vi "parseCommand.vi"(8 "error in (no error)":errorcluster, 10 "CMDString":string, 11 "CommandParser in":refnum<class "CommandParser.lvclass">) -> (0 "error out":errorcluster, 1 "parameter":variant, 2 "MonoCommand":T1, 3 "CommandParser out":refnum<class "CommandParser.lvclass">)   [LabVIEW 2020, in "CommandParser.lvclass"]
uses:
  CommandParser.lvclass
  Typedefs/MonoCommand.ctl
  Typedefs/wavelength.ctl
  Typedefs/slitWidth.ctl
  Typedefs/GratingType.ctl
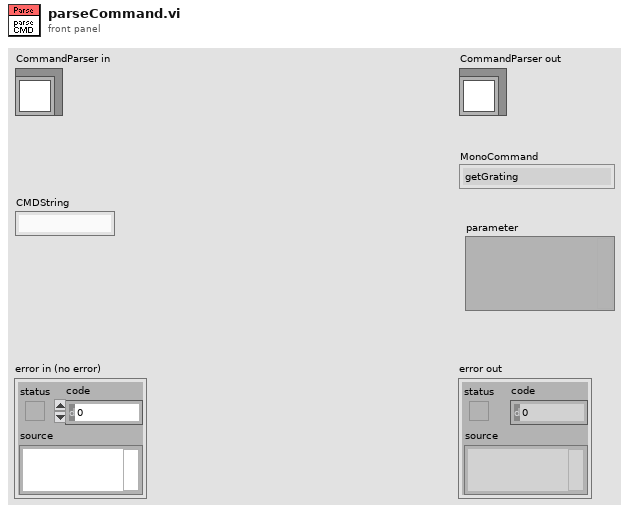
[diagram p1: front panel]
types:
  T1 = typedef "MonoCommand.ctl" = enum16{"getGrating", "getFrontEntranceSlitPosition", "getFrontExitSlitPosition", "getWavelength", "setWavelength", "setGrating", "setFrontEntranceSlitPosition", "setFrontExitSlitPosition", "calibrateWavelength", "getStatus", "Unknown", "reset", "setAll"}
  T2 = typedef "wavelength.ctl" = dbl
  T3 = typedef "slitWidth.ctl" = dbl
  T4 = typedef "GratingType.ctl" = enum16{"Blue", "Red", "Mirror"}
  T5 = cluster{"wavelength":T2, "frontExitSlitWidth":T3, "fronEntranceSlitWidth":T3, "GratingType":T4}
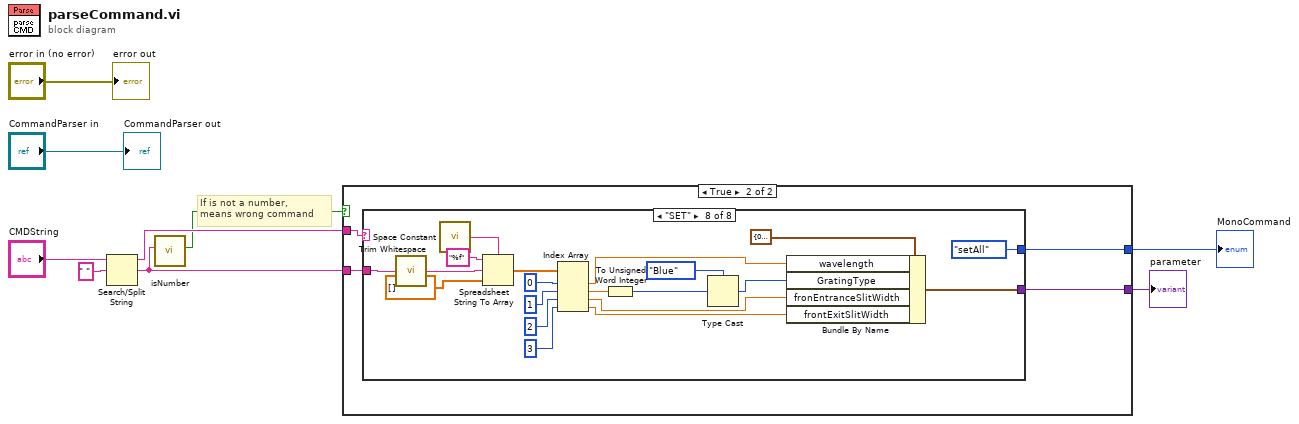
[diagram p0: block diagram]
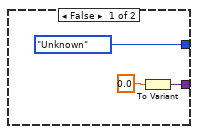
[diagram p2: hidden frame]
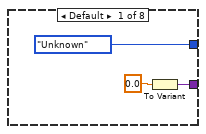
[diagram p3: hidden frame]
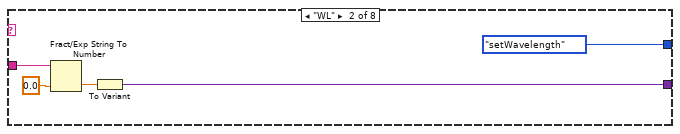
[diagram p4: hidden frame]
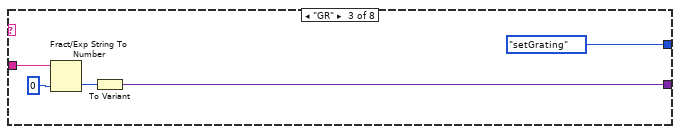
[diagram p5: hidden frame]
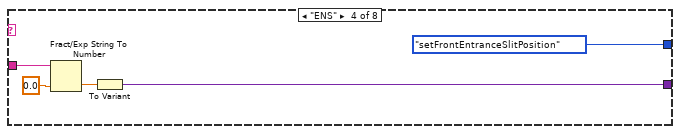
[diagram p6: hidden frame]
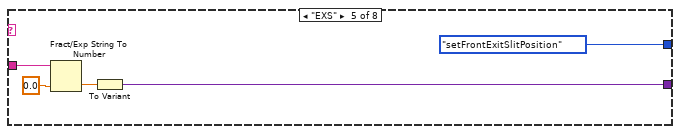
[diagram p7: hidden frame]
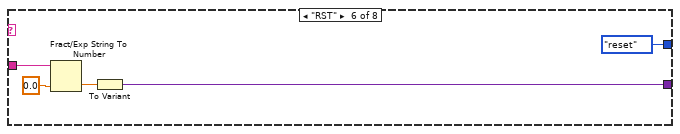
[diagram p8: hidden frame]
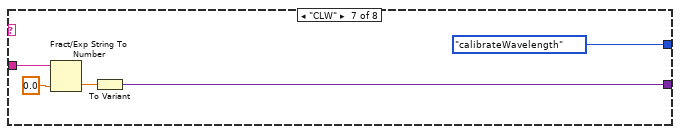
[diagram p9: hidden frame]
diagram:
  # "If is not a number, \nmeans wrong command"
  n1 = Search/Split String(string="CMDString", search string/char (-)=" ") -> (substring before match=w3:string, match + rest of string=w2:string)  [unwired: 1 in, 1 out]
  n2 = call "isNumber.vi"("string"=w2) -> ("isNumber?"=w1:bool)  [unwired: 8 in, 2 out]
  n3 = case shown="True" w1 {
    tunnel: [MonoCommand."Unknown" ("MonoCommand") w16] -> w6
    tunnel: w3 -> [_ w15]
    tunnel: [w11 w14] -> w5
    tunnel: w2 -> [_ w13]
    frame False {
      n4 = To Variant(anything=T2 0.0 ("wavelength")) -> (Variant=w11:variant)
    }
    frame True {
      n5 = case shown="\"SET\"" w15 {
        tunnel: [MonoCommand."Unknown" ("MonoCommand") MonoCommand."setWavelength" ("MonoCommand") MonoCommand."setGrating" ("MonoCommand") MonoCommand."setFrontEntranceSlitPosition" ("MonoCommand") MonoCommand."setFrontExitSlitPosition" ("MonoCommand") MonoCommand."reset" ("MonoCommand") MonoCommand."calibrateWavelength" ("MonoCommand") MonoCommand."setAll" ("MonoCommand")] -> w16
        tunnel: w13 -> [_ w24 w29 w33 w36 w41 w49 w51]
        tunnel: [w17 w22 w25 w34 w37 w40 w46 w52] -> w14
        frame Default {
          n6 = To Variant(anything=T2 0.0 ("wavelength")) -> (Variant=w17:variant)
        }
        frame "WL" {
          n7 = Fract/Exp String To Number(string=w24, default (0 dbl)=T2 0.0 ("wavelength")) -> (number=w20:dbl)  [unwired: 2 in, 1 out]
          n8 = To Variant(anything=w20) -> (Variant=w22:variant)
        }
        frame "GR" {
          n9 = Fract/Exp String To Number(string=w29, default (0 dbl)=u16 0) -> (number=w26:u16)  [unwired: 2 in, 1 out]
          n10 = To Variant(anything=w26) -> (Variant=w25:variant)
        }
        frame "ENS" {
          n11 = Fract/Exp String To Number(string=w33, default (0 dbl)=T3 0.0 ("position")) -> (number=w32:dbl)  [unwired: 2 in, 1 out]
          n12 = To Variant(anything=w32) -> (Variant=w34:variant)
        }
        frame "EXS" {
          n13 = Fract/Exp String To Number(string=w36, default (0 dbl)=T3 0.0 ("position")) -> (number=w38:dbl)  [unwired: 2 in, 1 out]
          n14 = To Variant(anything=w38) -> (Variant=w37:variant)
        }
        frame "RST" {
          n15 = Fract/Exp String To Number(string=w41, default (0 dbl)=T3 0.0 ("position")) -> (number=w42:dbl)  [unwired: 2 in, 1 out]
          n16 = To Variant(anything=w42) -> (Variant=w40:variant)
        }
        frame "CLW" {
          n17 = Fract/Exp String To Number(string=w49, default (0 dbl)=T2 0.0 ("wavelength")) -> (number=w45:dbl)  [unwired: 2 in, 1 out]
          n18 = To Variant(anything=w45) -> (Variant=w46:variant)
        }
        frame "SET" {
          n19 = call <vilib>:"Trim Whitespace.vi"("string"=w51) -> ("trimmed string"=w50:string)  [unwired: 1 in]
          n20 = call <vilib>:"Space Constant.vi"() -> ("String"=w67:string)
          n21 = Spreadsheet String To Array(delimiter (Tab)=w67, format string="%f", spreadsheet string=w50, array type (2D Dbl)=dbl[] []) -> (array=w53:dbl[])
          n22 = Index Array(array=w53, index #1=0 ("index"), index #2=1 ("index"), index #3=2 ("index"), index #4=3 ("index")) -> (element #1=w59:dbl, element #2=w62:dbl, element #3=w60:dbl, element #4=w61:dbl)
          n23 = To Unsigned Word Integer(number=w62) -> (unsigned 16bit integer=w63:u16)
          n24 = Type Cast(type=GratingType."Blue" ("GratingType"), x=w63) -> (*(type *) &x=w64:T4)
          n25 = Bundle By Name(cluster=T5 {"wavelength"=0.0, "frontExitSlitWidth"=0.0, "fronEntranceSlitWidth"=0.0, "GratingType"=enum."Blue"} ("Cluster"), "wavelength"=w59, "GratingType"=w64, "fronEntranceSlitWidth"=w60, "frontExitSlitWidth"=w61) -> (w52:T5)
        }
      }
    }
  }
  "MonoCommand" <- w6
  "parameter" <- w5
  "error out" <- "error in (no error)"
  "CommandParser out" <- "CommandParser in"
